vi "Test Actor Trace Generation.vi"(11 "Test Case In":refnum<class "AF Test.lvclass">) -> (0 "error out":errorcluster, 3 "Test Case Out":refnum<class "AF Test.lvclass">)   [LabVIEW 2020, in "AF Test.lvclass"]
uses:
  AF Test.lvclass
  C:/Program Files (x86)/National Instruments/LabVIEW 2020/vi.lib/Astemes/LUnit/Test Case.lvclass
  <vilib>/Astemes/LUnit/Test Case.lvclass/Test Case.ctl
  4993e8ee-a06a-463a-9684-69129f64d5ce.vi
  <vilib>/Astemes/LUnit/Core/LUnit Test Case/Private/Append Pass Result.vi
  <vilib>/Astemes/LUnit/Core/LUnit Test Case/Private/Append Fail Result.vi
  4993e8ee-a06a-463a-9684-69129f64d5ce.vi/9c5d11cd-9439-4240-a1ee-d9baace9c924.vi
  <vilib>/Astemes/LUnit/Core/LUnit Test Case/Private/Run In UI.vi
  <vilib>/Utility/error.llb/Clear Errors.vi
  AF Test.lvclass/AF Test.ctl
  ActorFramework/Actor/Actor.lvclass
  Test Harness/AF Trace Queue/AF Trace Queue.lvclass
  ActorFramework/Stop Msg/Stop Msg.lvclass
panel:
  out "Array":string[](array[string])
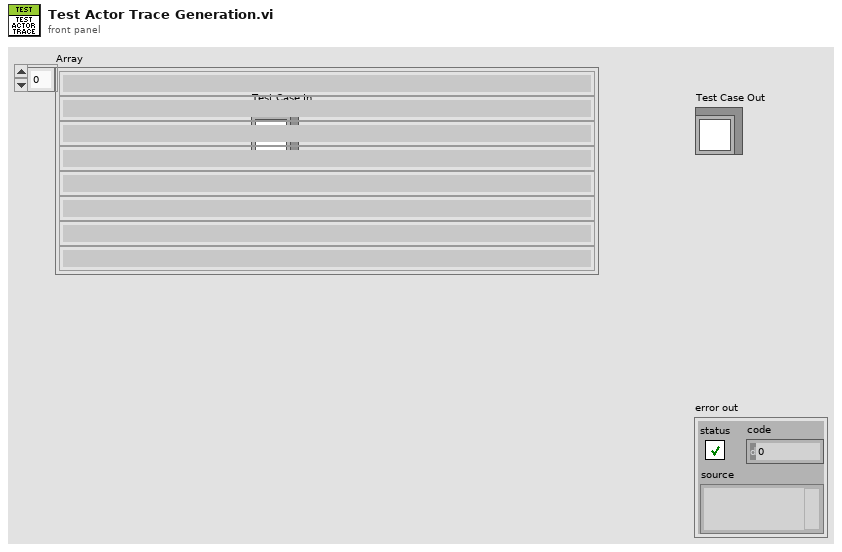
[diagram p1: front panel]
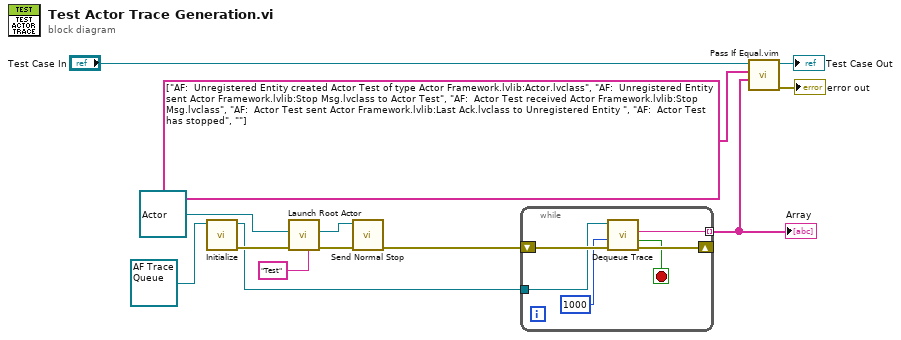
[diagram p0: block diagram]
diagram:
  n1 = call-dynamic "Initialize.vi"("AF Trace Queue in"=refnum<class "AF Trace Queue.lvclass"> refnum) -> ("error out"=w9:errorcluster, "AF Trace Queue out"=w5:refnum<class "AF Trace Queue.lvclass">)  [unwired: 9 in]
  n2 = call "Launch Root Actor.vi"("Debug Alias"="Test", "error in (no error)"=w9, "Actor"=refnum<class "Actor.lvclass"> refnum ("Actor Framework:Actor")) -> ("error out"=w8:errorcluster, "Actor's Enqueuer"=w6:refnum<class "Message Enqueuer.lvclass">)  [unwired: 7 in]
  n3 = call "Send Normal Stop.vi"("error in (no error)"=w8, "Message Enqueuer"=w6) -> ("error out"=w7:errorcluster)  [unwired: 9 in]
  n4 = while {
    tunnel: w5 -> [w18]
    shift-right: [w17] -> _
    shift-left: w7 -> [w19]
    tunnel: [w14] -> w1 mode=indexing
    stop <- w15 stop-if-true
    n5 = call "Dequeue Trace.vi"("error in (no error)"=w19, "timeout in ms (-1)"=1000, "AF Trace Queue in"=w18) -> ("error out"=w17:errorcluster, "timed out?"=w15:bool, "Trace String"=w14:string)  [unwired: 5 in, 1 out]
  }
  "Array" <- w1
  n6 = call "Pass If Equal.vim"("Actual"=w1, "Expected"=string[] ["AF:  Unregistered Entity created Actor Test of type Actor Framework.lvlib:Actor.lvclass", "AF:  Unregistered Entity sent Actor Framework.lvlib:Stop Msg.lvclass to Actor Test", "AF:  Actor Test received Actor Framework.lvlib:Stop Msg.lvclass", "AF:  Actor Test sent Actor Framework.lvlib:Last Ack.lvclass to Unregistered Entity ", "AF:  Actor Test has stopped", ""] ("Array"), "LUnit Test Case In"="Test Case In") -> ("error out"=→"error out":errorcluster, "LUnit Test Case Out"=→"Test Case Out":refnum<class "AF Test.lvclass">)  [unwired: 7 in]
